vi "util-daily-seconds.vi"(11 "seconds since 1Jan1904":timestamp) -> (3 "Numeric":i32)   [LabVIEW 2024]
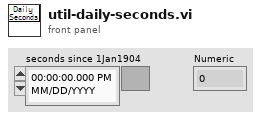
[diagram p1: front panel]
types:
  T1 = typedef "LVDateTimeRec.ctl" = cluster{"fractional second":dbl, "second":i32, "minute":i32, "hour":i32, "day of month":i32, "month":i32, "year":i32, "day of week":i32, "day of year":i32, "DST":i32}
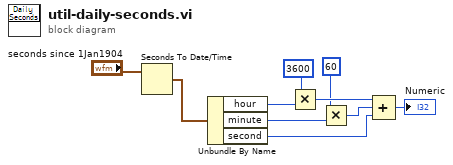
[diagram p0: block diagram]
diagram:
  n1 = Seconds To Date/Time(time stamp (now)="seconds since 1Jan1904") -> (date time rec=w2:T1)  [unwired: 1 in]
  n2 = Unbundle By Name(w2) -> ("hour"=w3:i32, "minute"=w5:i32, "second"=w9:i32)
  n3 = Multiply(x=3600, y=w3) -> (x*y=w7:i32)
  n4 = Multiply(x=60, y=w5) -> (x*y=w8:i32)
  n5 = Compound Arithmetic op=ADD(w7, w8, w9) -> (→"Numeric":i32)
